vi "Upload Record (F64).vi"(0 "Instrument Handle In":i32, 1 "Count":i32, 2 "Time Interval":dbl, 3 "Time Offset":dbl, 5 "Ref Channel":i32(ring) caption="Channel" items=["Calc Channel 1", "Calc Channel 2", "Calc Channel 3", "Calc Channel 4", "Ref Channel 1", "Ref Channel 2", "Ref Channel 3", "Ref Channel 4"], 7 "Type":i32, 9 "Points":u32, 11 "error in":errorcluster, 12 "Waveform":dbl[](array[numeric]), 13 "Voltage Interval":dbl, 14 "Voltage Offset":dbl) -> (4 "Instrument Handle Out":i32, 15 "error out":errorcluster)   [LabVIEW 8.6, in "ZTScopeM.lvlib"]
doc: "Read the waveform in the source channel. The returned data format depends on the Transfer Type. Use \"Read Waveform Preamble\" to get the appropriate time and magnitude bases."
uses:
  ZTScopeM.lvlib
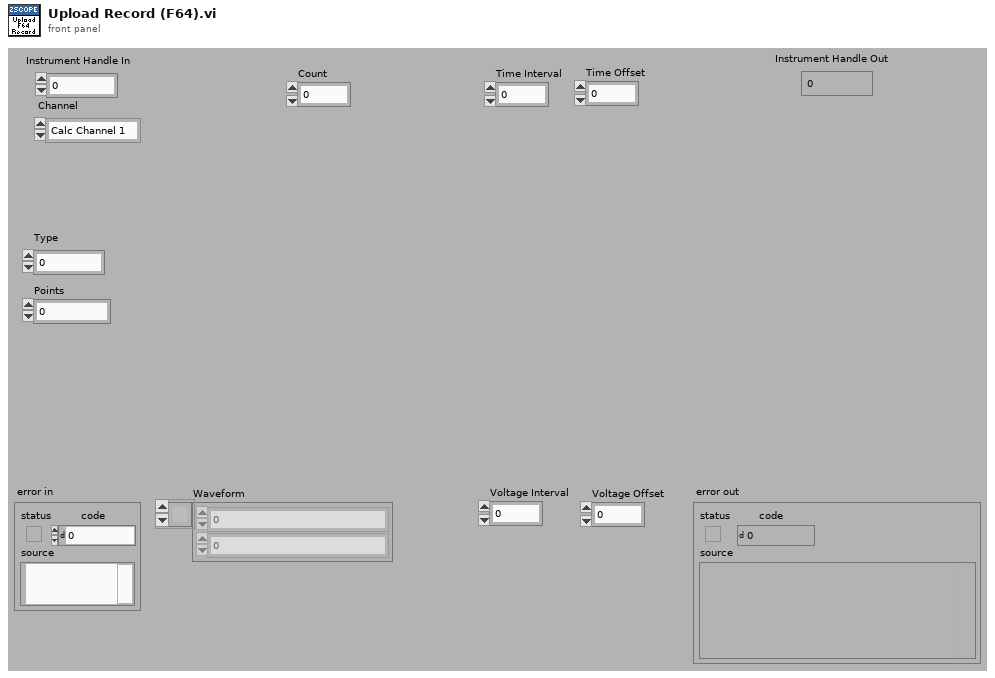
[diagram p1: front panel]
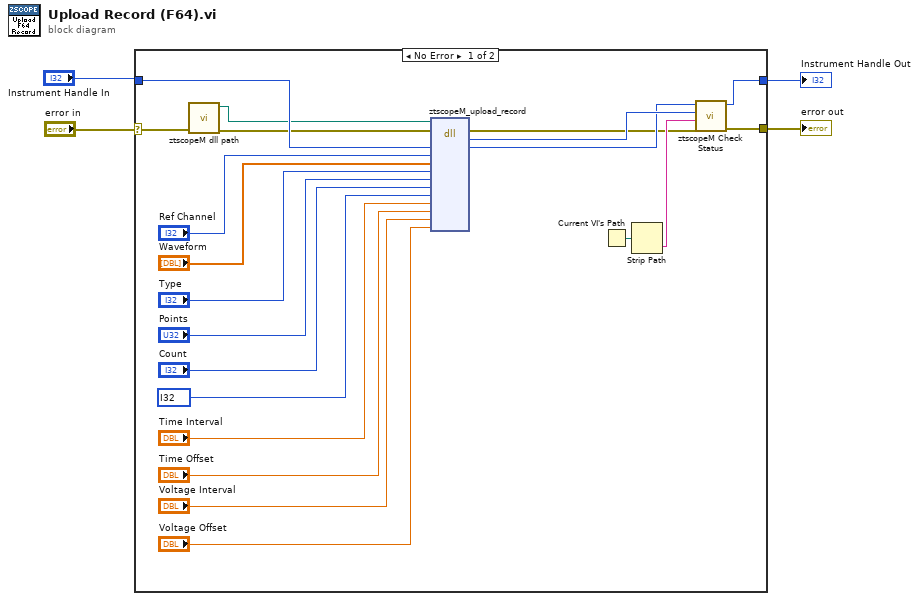
[diagram p0: block diagram]
diagram:
  n1 = case shown="No Error" "error in" {
    selector: "error in" -> [w17 w27]
    tunnel: [w20 w27] -> w1
    tunnel: "Instrument Handle In" -> [w19 w26]
    tunnel: [w21 w26] -> w3
    frame #0 {
      w12 = i32 ? items=["s8", "s16", "s32", "f32", "f64"] ("Transfer Type")
      n2 = call "ztscopeM dll path.vi"("error in (no error)"=w17) -> ("error out"=w6:errorcluster, "<instrument>.dll path"=w16:path)  [unwired: 9 in]
      n3 = dll-call lib="C:/Projects/codedepot/Teradyne/2016-1034 Teradyne ZScope API/Software/Validation/C/bin/ztscopeM Log3.dll" fn="ztscopeM_upload_record"(path in=w16, error in=w6, "instrumentHandle"=w19, "ref_channel"="Ref Channel", "Waveform"="Waveform", "type"="Type", "points"="Points", "count"="Count", "transferType"=w12, "time_interval"="Time Interval", "time_offset"="Time Offset", "voltage_interval"="Voltage Interval", "voltage_offset"="Voltage Offset") -> (error out=w5:errorcluster, "return type"=w23:i32, "instrumentHandle"=w22:i32)  [unwired: 11 in, 1 out]
      n4 = Current VI's Path() -> (path=w25:path)
      n5 = Strip Path(path=w25) -> (name=w24:string)  [unwired: 1 out]
      n6 = call "ztscopeM Check Status.vi"("error in"=w5, "name of VI"=w24, "status (return code)"=w23, "instrument handle in"=w22) -> ("error out"=w20:errorcluster, "instrument handle out"=w21:i32)  [unwired: 2 in]
    }
    frame #1 {
    }
  }
  "Instrument Handle Out" <- w3
  "error out" <- w1
